vi "Setup AI.vi"(0 "reference in":refnum<class "AI.lvclass">, 1 "AI Units":i32(ring)=10348 items=["Volts"=10348, "From Custom Scale"=10065], 3 "AI Physical Input Configuration":i32(ring)=10106 items=["Default"=-1, "RSE"=10083, "NRSE"=10078, "Differential"=10106, "Pseudodifferential"=12529], 4 "AI Module Names (NI-Max Name)":string[](array[string])=["AI-32CH"], 5 "Number of Channels Per AI  Module":i32[](array[numeric])=[8], 7 "error in (no error)":errorcluster, 12 "Number of AI Samples Per Channel":i32=1000, 13 "AI Minimum Voltage Value":dbl=-5.0 format="%0.2f", 15 "AI Maximum Voltage Value":dbl=5.0 format="%0.2f", 17 "Linear Scale Slope":dbl=1.0 format="%0.2f", 19 "Linear Scale Y-Intercept":dbl format="%0.2f") -> (20 "reference out":refnum<class "AI.lvclass">, 27 "error out":errorcluster)   [LabVIEW 2017, in "AI.lvclass"]
uses:
  AI.lvclass
  <vilib>/DAQmx/create/scale.llb/DAQmx Create Scale (Linear).vi
  <vilib>/DAQmx/create/channels.llb/DAQmx Create Channel (AI-Voltage-Basic).vi
  <vilib>/DAQmx/configure/timing.llb/DAQmx Timing (Sample Clock).vi
  <resource>/objmgr/daqmx.rc
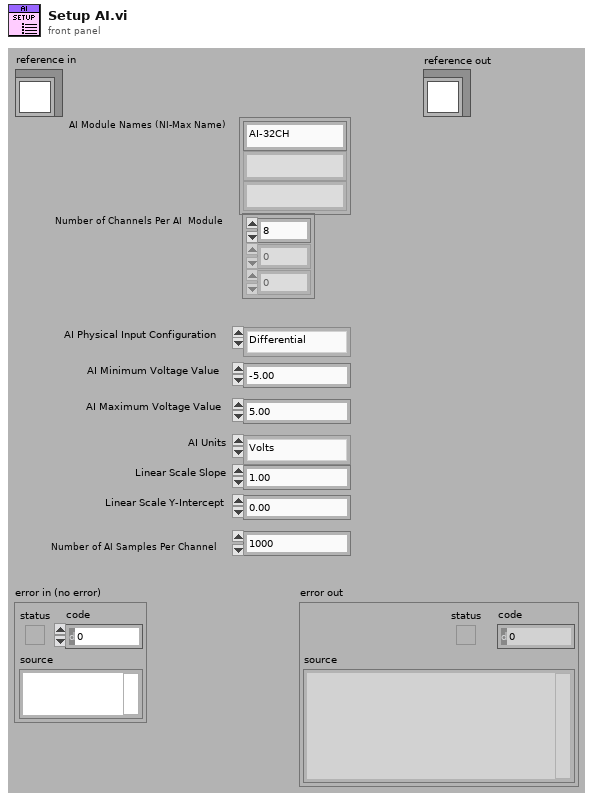
[diagram p1: front panel]
types:
  T1 = typedef "AI.lvclass/ObjectAttributes.ctl" = cluster{"AI Task":refnum<k21>, "AI On/Off Status":bool, "AI Sampling Rate (Samples/Seconds)":u32, "Number of AI Samples Per Channel":i32, "AI Voltage Range":u8, "AI Readings":dbl[][], "Number of AI Modules":i32, "Number of Total AI Channels":i32, "AI Module Names (NI-Max Name)":string[], "Number of Channels Per AI  Module":i32[], "AI VI Reference":refnum<vi>}
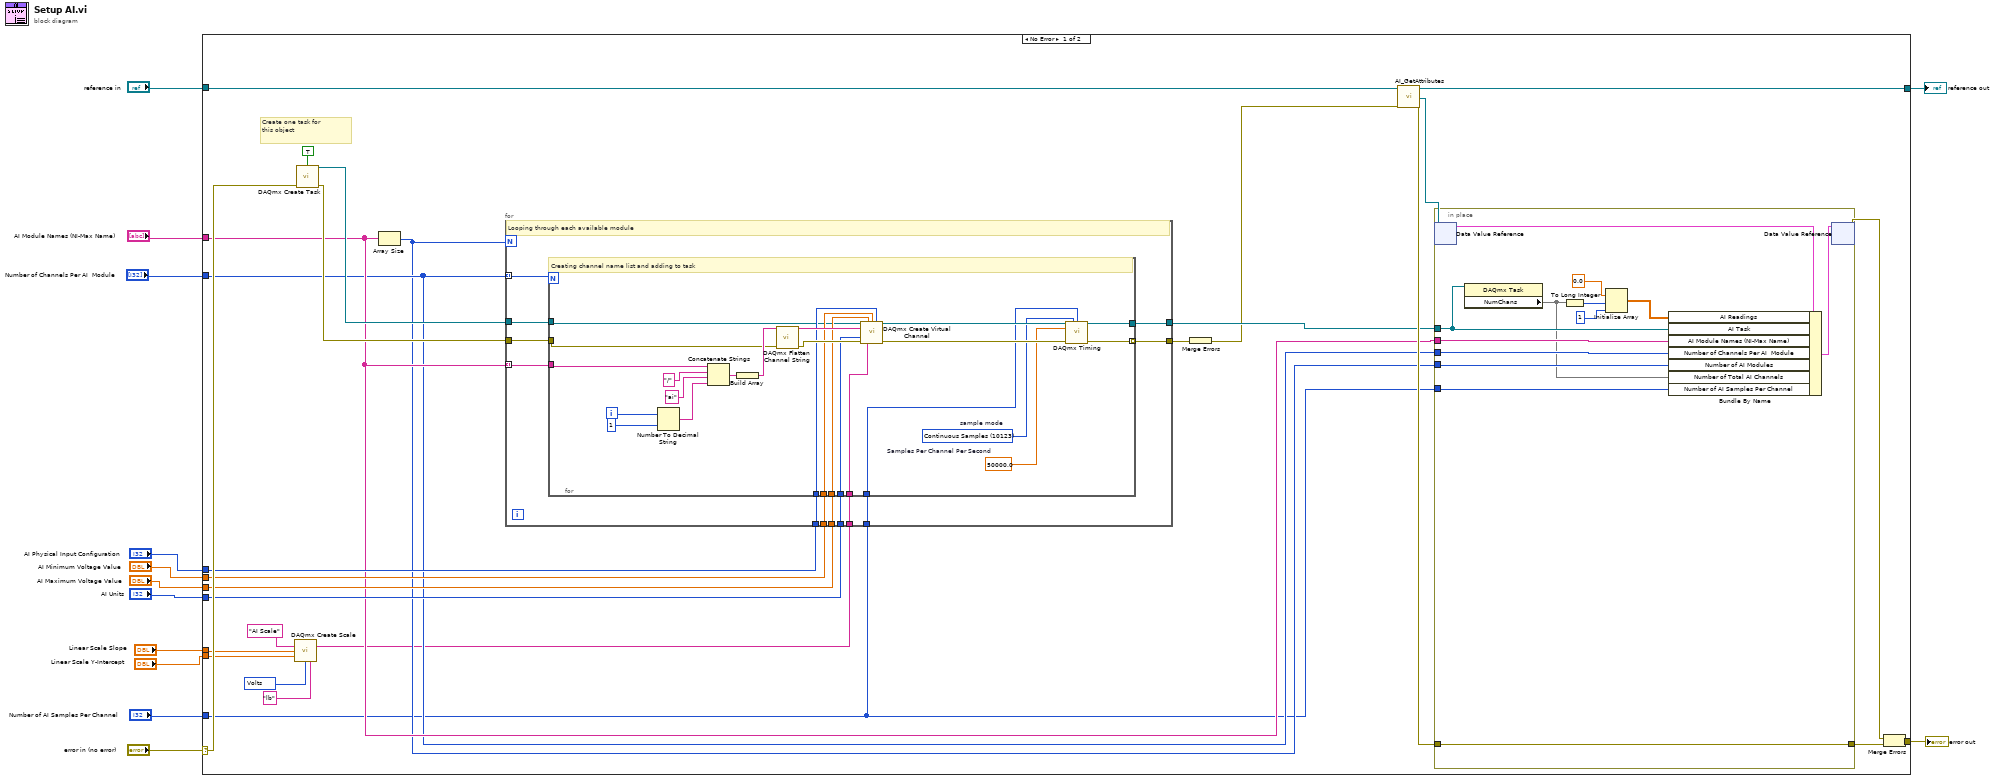
[diagram p0: block diagram]
diagram:
  n1 = case shown="No Error" "error in (no error)" {
    selector: "error in (no error)" -> [w33 w92]
    tunnel: [w38 w92] -> w12
    tunnel: [w39 w91] -> w10
    tunnel: "reference in" -> [w41 w91]
    tunnel: "AI Module Names (NI-Max Name)" -> [w23 _]
    tunnel: "Number of Channels Per AI  Module" -> [w22 _]
    tunnel: "AI Physical Input Configuration" -> [w30 _]
    tunnel: "AI Minimum Voltage Value" -> [w29 _]
    tunnel: "AI Maximum Voltage Value" -> [w28 _]
    tunnel: "AI Units" -> [w27 _]
    tunnel: "Number of AI Samples Per Channel" -> [w20 _]
    tunnel: "Linear Scale Slope" -> [w17 _]
    tunnel: "Linear Scale Y-Intercept" -> [w16 _]
    frame No Error {
      w15 = 10348 items=["Volts"=10348, "Amps"=10342, "Deg F"=10144, "Deg C"=10143, "Deg R"=10145, "Kelvins"=10325, "Strain"=10299, "Ohms"=10384, "Hz"=10373, "Seconds"=10364, "Meters"=10219, "Inches"=10379, "Degrees"=10146, "Radians"=10273, "Ticks"=10304, "g"=10186, "m/s^2"=12470, "m/s"=15959, "in/s"=15960, "Pascals"=10081, "Newtons"=15875, "Pounds"=15876, "kgf"=15877, "psi"=15879, "bar"=15880, "Nm"=15881, "oz-in"=15882, "lb-in"=15883, "lb-ft"=15884, "Volts/Volt"=15896, "mVolts/Volt"=15897, "pCoulombs"=16103, "Coulombs"=16102, "From TEDS"=12516] ("pre-scaled units")
      # "Create one task for \nthis object"
      n2 = call-poly <vilib>:"DAQmx Create Scale.vi"("name"="AI Scale", "slope"=w17, "y-intercept"=w16, "pre-scaled units"=w15, "scaled units"="lb") -> ("scale out"=w18:tag)  [unwired: 9 in, 1 out]
      n3 = call <vilib>:"DAQmx Create Task.vi"("auto cleanup"=TRUE, "error in"=w33) -> ("task out"=w32:refnum<k21>, "error out"=w31:errorcluster)  [unwired: 12 in]
      n4 = Array Size(array=w23) -> (size(s)=w21:i32)
      n5 = for {
        N: w21 -> [_]
        tunnel: [w53] -> w25
        tunnel: [w52] -> w26
        tunnel: w22 -> [w51] mode=indexing
        tunnel: w32 -> [w50]
        tunnel: w31 -> [w49]
        tunnel: w23 -> [w48] mode=indexing
        tunnel: w30 -> [w47]
        tunnel: w29 -> [w46]
        tunnel: w28 -> [w45]
        tunnel: w27 -> [w44]
        tunnel: w20 -> [w43]
        tunnel: w18 -> [w42]
        # "Looping through each available module"
        n6 = for {
          N: w51 -> [_]
          tunnel: [w67] -> w52
          tunnel: [w65] -> w53 mode=indexing
          tunnel: w50 -> [w56]
          tunnel: w49 -> [w62]
          tunnel: w48 -> [w61]
          tunnel: w44 -> [w60]
          tunnel: w45 -> [w59]
          tunnel: w46 -> [w58]
          tunnel: w47 -> [w57]
          tunnel: w43 -> [w55]
          tunnel: w42 -> [w54]
          i -> [w77]
          w63 = 10123 items=["Finite Samples"=10178, "Continuous Samples"=10123, "Hardware Timed Single Point"=12522]  # sample mode
          w64 = 50000.0  # Samples Per Channel Per Second
          # "Creating channel name list and adding to task"
          n7 = Number To Decimal String(number=w77, width (-)=i16 1) -> (decimal integer string=w74:string)
          n8 = Concatenate Strings(w61, "/", "ai", w74) -> (w71:string)
          n9 = Build Array(w71) -> (w70:string[])
          n10 = call <vilib>:"DAQmx Flatten Channel String.vi"("names in"=w70, "error in"=w62) -> ("names out"=w72:string, "error out"=w73:errorcluster)  [unwired: 12 in]
          n11 = call-poly <vilib>:"DAQmx Create Virtual Channel.vi"("task in"=w56, "maximum value"=w59, "minimum value"=w58, "input terminal configuration"=w57, "physical channels"=w72, "units"=w60, "error in"=w73, "custom scale name"=w54) -> ("task out"=w68:refnum<k21>, "error out"=w66:errorcluster)  [unwired: 6 in]
          n12 = call-poly <vilib>:"DAQmx Timing.vi"("task/channels in"=w68, "sample mode"=w63, "samples per channel"=w55, "rate"=w64, "error in"=w66) -> ("task out"=w67:refnum<k21>, "error out"=w65:errorcluster)  [unwired: 9 in]
        }
      }
      n13 = Merge Errors(w25) -> (w24:errorcluster)
      n14 = call "AI_GetAttributes.vi"("reference in"=w41, "error in (no error)"=w24) -> ("reference out"=w39:refnum<class "AI.lvclass">, "DataRef"=w37:refnum<data-value>, "error out"=w36:errorcluster)  [unwired: 14 in, 1 out]
      n15 = in-place {
        in-place-border: w36 -> [w88]
        in-place-border: [w88] -> w35
        in-place-border: w26 -> [w84]
        in-place-border: w23 -> [w87]
        in-place-border: w22 -> [w86]
        in-place-border: w21 -> [w85]
        in-place-border: w20 -> [w78]
        n16 = in-place-dvr #1(w37) -> (w89:T1)  [unwired: 1 out]
        n17 = property class="DAQmx Task"(reference=w84) -> ("NumChans"=w79)  [unwired: 1 in, 2 out]
        n18 = To Long Integer(number=w79) -> (32bit integer=w83:i32)
        n19 = Initialize Array(0.0, w83, 1 ("dimension size")) -> (w82:dbl[][])
        n20 = Bundle By Name(cluster=w89, "AI Readings"=w82, "AI Task"=w84, "AI Module Names (NI-Max Name)"=w87, "Number of Channels Per AI  Module"=w86, "Number of AI Modules"=w85, "Number of Total AI Channels"=w79, "Number of AI Samples Per Channel"=w78) -> (w90:T1)
        n21 = in-place-dvr #1(w90) -> (w40:errorcluster)  [unwired: 1 out]
      }
      n22 = Merge Errors(w40, w35) -> (w38:errorcluster)
    }
    frame Error {
    }
  }
  "error out" <- w12
  "reference out" <- w10
